vi "tm3samp_dcimgrecorder.vi"() -> ()   [LabVIEW 2011]
panel:
  out "Frames Recorded":i32
  in  "DCIMG Path":path
  in  "Frames":i32=100
  out "Error Out":errorcluster
  # "This is an example of how to use the\nhard disk recorder functions to record\nimages to a DCIMG file."
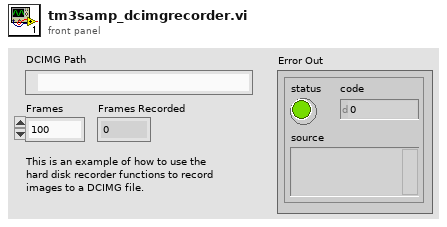
[diagram p1: front panel]
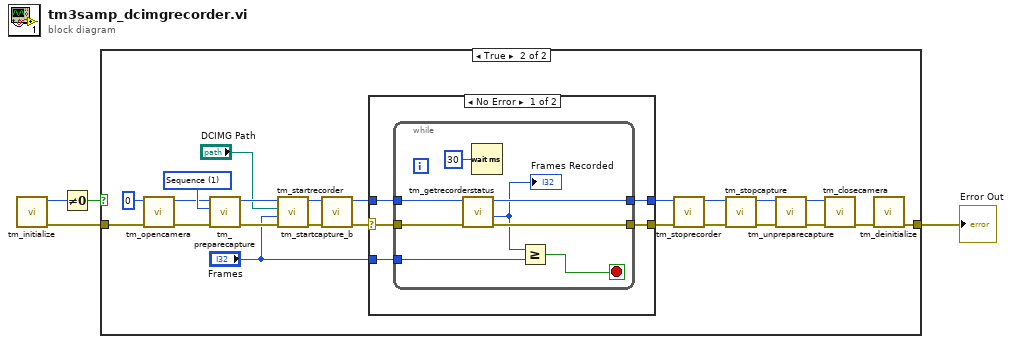
[diagram p0: block diagram]
diagram:
  n1 = call <userlib>:"tm_initialize.vi"() -> ("error out"=w1:errorcluster, "Number Of Cameras"=w2:u32)  [unwired: 10 in]
  n2 = Not Equal To 0?(x=w2) -> (x != 0?=w4:bool)
  n3 = case shown="True" w4 {
    tunnel: w1 -> [w5 w28]
    tunnel: [w5 w24] -> w3
    frame False {
    }
    frame True {
      w26 = 1 items=["Snap", "Sequence"] ("Capture mode")
      n4 = call <userlib>:"tm_opencamera.vi"("error in (no error)"=w28, "Camera Index"=u32 0) -> ("error out"=w12:errorcluster, "Handle out"=w13:u32)  [unwired: 8 in]
      n5 = call <userlib>:"tm_preparecapture.vi"("error in (no error)"=w12, "Capture mode"=w26, "Handle in"=w13) -> ("error out"=w21:errorcluster, "Handle out"=w20:u32)  [unwired: 5 in, 2 out]
      n6 = call <userlib>:"tm_startrecorder.vi"("error in (no error)"=w21, "frames"="Frames", "File"="DCIMG Path", "Handle in"=w20) -> ("error out"=w19:errorcluster, "Handle out"=w18:u32)  [unwired: 6 in]
      n7 = call <userlib>:"tm_startcapture_b.vi"("error in (no error)"=w19, "Handle in"=w18) -> ("error out"=w17:errorcluster, "Handle out"=w16:u32)  [unwired: 8 in]
      n8 = case shown="No Error" w17 {
        selector: w17 -> [w33 w42]
        tunnel: w16 -> [w32 w43]
        tunnel: [w30 w43] -> w6
        tunnel: [w31 w42] -> w7
        tunnel: "Frames" -> [w29 _]
        frame No Error {
          n9 = while {
            tunnel: w33 -> [w39]
            tunnel: w32 -> [w38]
            tunnel: [w37] -> w31
            tunnel: [w40] -> w30
            tunnel: w29 -> [w41]
            stop <- w35 stop-if-true
            n10 = call <userlib>:"tm_getrecorderstatus.vi"("error in (no error)"=w39, "Handle"=w38) -> ("error out"=w37:errorcluster, "Count"=w36:i32, "Handle"=w40:u32)  [unwired: 6 in, 1 out]
            "Frames Recorded" <- w36
            n11 = Wait (ms)(milliseconds to wait=u32 30) -> ()  [unwired: 1 out]
            n12 = Greater Or Equal?(x=w36, y=w41) -> (x >= y?=w35:bool)
          }
        }
        frame Error {
        }
      }
      n13 = call <userlib>:"tm_stoprecorder.vi"("error in (no error)"=w7, "Handle in"=w6) -> ("error out"=w8:errorcluster, "Handle out"=w9:u32)  [unwired: 8 in]
      n14 = call <userlib>:"tm_stopcapture.vi"("error in (no error)"=w8, "Handle in"=w9) -> ("error out"=w11:errorcluster, "Handle out"=w10:u32)  [unwired: 8 in]
      n15 = call <userlib>:"tm_unpreparecapture.vi"("error in (no error)"=w11, "Handle in"=w10) -> ("error out"=w23:errorcluster, "Handle out"=w22:u32)  [unwired: 8 in]
      n16 = call <userlib>:"tm_closecamera.vi"("error in (no error)"=w23, "Handle in"=w22) -> ("error out"=w25:errorcluster)  [unwired: 9 in]
      n17 = call <userlib>:"tm_deinitialize.vi"("error in (no error)"=w25) -> ("error out"=w24:errorcluster)  [unwired: 10 in]
    }
  }
  "Error Out" <- w3
